vi "Time.vi"(8 "error in (no error)":errorcluster, 10 "Control In":T1={"I-O.lvclass"=refnum, "Gantry"=refnum, "Dispenser"="COM1"}, 11 "Sensor Dispense in":refnum<class "Sensor Dispense.lvclass">) -> (0 "error out":errorcluster, 1 "Timing Data":i32[](array[numeric]), 2 "Control Out":T1={"I-O.lvclass"=refnum, "Gantry"=refnum, "Dispenser"="COM1"}, 3 "Sensor Dispense out":refnum<class "Sensor Dispense.lvclass">)   [LabVIEW 2020, in "Sensor Dispense.lvclass"]
uses:
  Projects/Sensor Dispense.lvclass
  C:/Users/HEP/Documents/GitHub/UCSB-Gantry-HEP/Classes/Routine/Dispense/Dispense.lvclass
  Controller/Controllers.ctl
  Controller/I-O/I-O.lvclass
  C:/Program Files (x86)/Aerotech/A3200/LabVIEW/2010/Bin/Aerotech.A3200.dll
  Program Files (x86)/Aerotech/A3200/LabVIEW/2010/Bin/Aerotech.A3200.dll
  Projects/Sensor Dispense.lvclass/Sensor Dispense.ctl
  Controller/Motion/Motion.lvclass
  Controller/Motion/A3200/A3200.lvclass
  Controller/Controller.lvclass
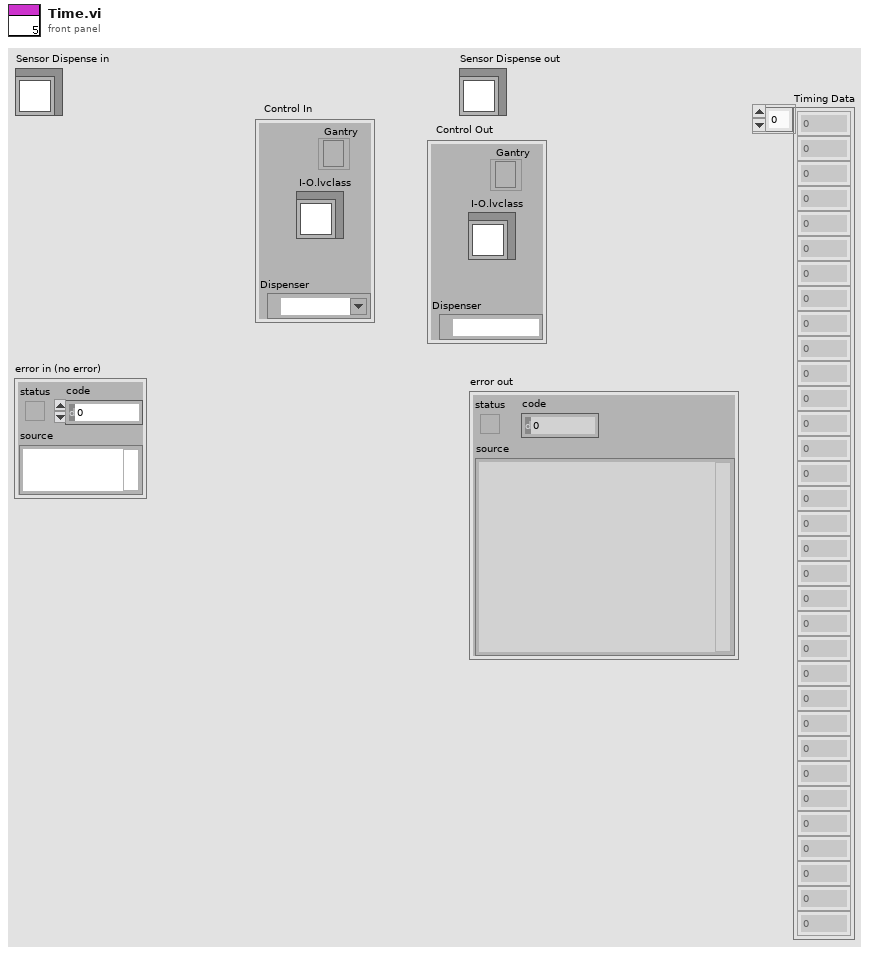
[diagram p1: front panel]
types:
  T1 = typedef "Controller.lvclass/Controllers.ctl" = cluster{"I-O.lvclass":refnum<class "I-O.lvclass">, "Gantry":refnum<k24>, "Dispenser":refnum<visa-resource-name>}
  T2 = cluster{"Endpoints":dbl[][], "Center":dbl[], "CW/CCW":dbl, "Dispense Type":enum16{"N-gon", "Square", "Arc", "Dot", "Line", "Circle"}}[]
  T3 = enum16{"N-gon", "Square", "Arc", "Dot", "Line", "Circle"}
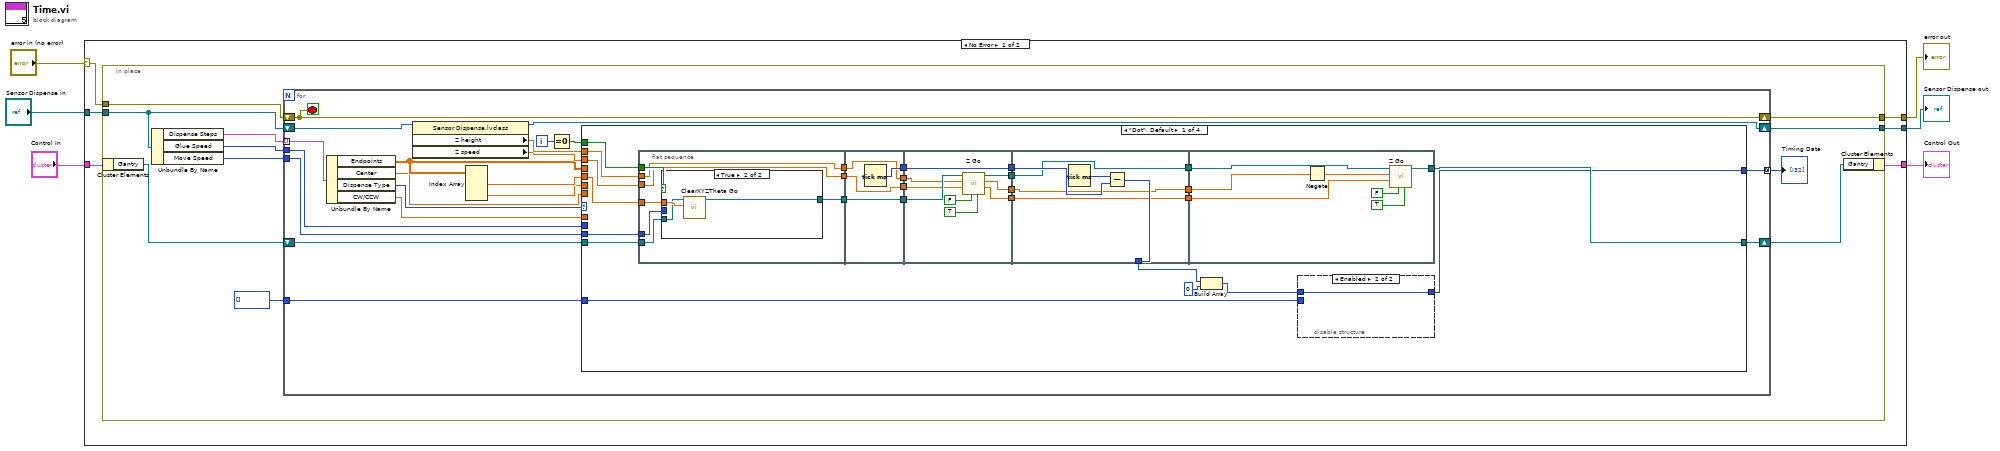
[diagram p0: block diagram]
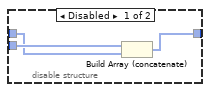
[diagram p2: hidden frame]
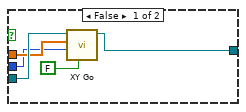
[diagram p3: hidden frame]
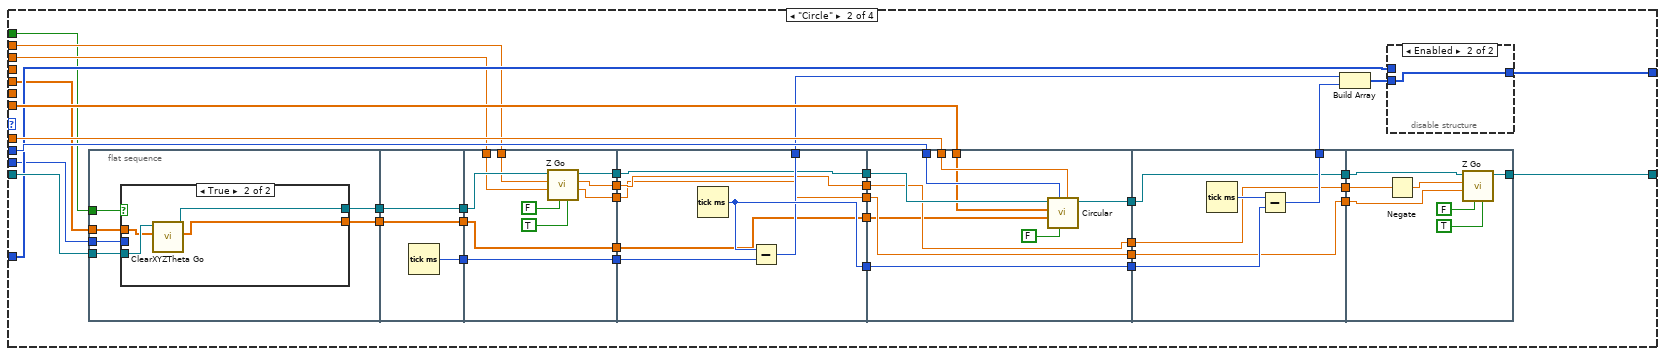
[diagram p4: hidden frame]
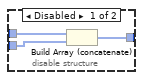
[diagram p5: hidden frame]
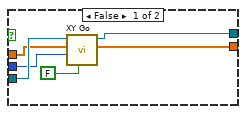
[diagram p6: hidden frame]
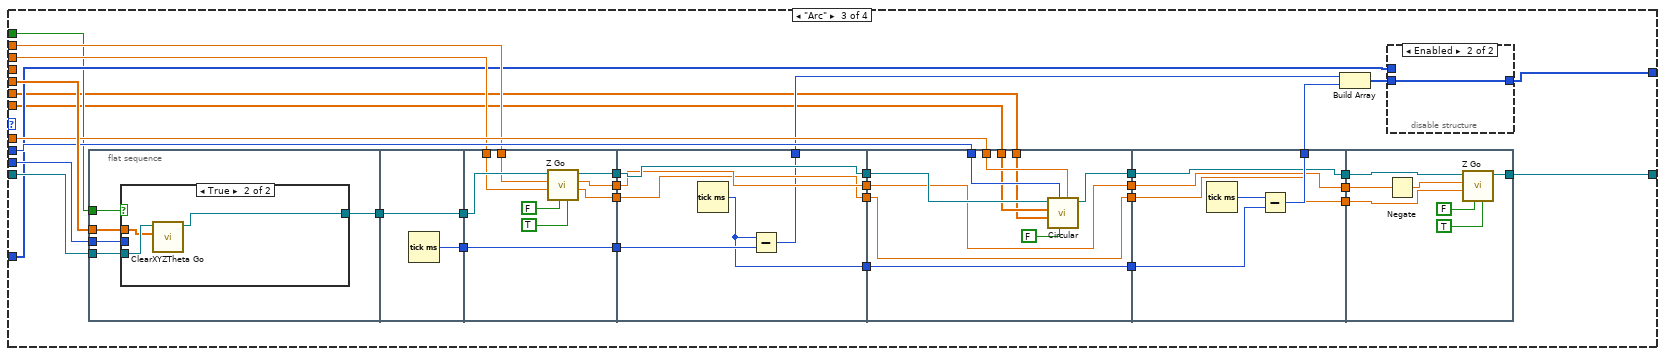
[diagram p7: hidden frame]
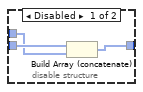
[diagram p8: hidden frame]
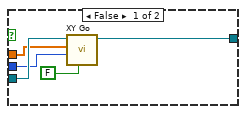
[diagram p9: hidden frame]
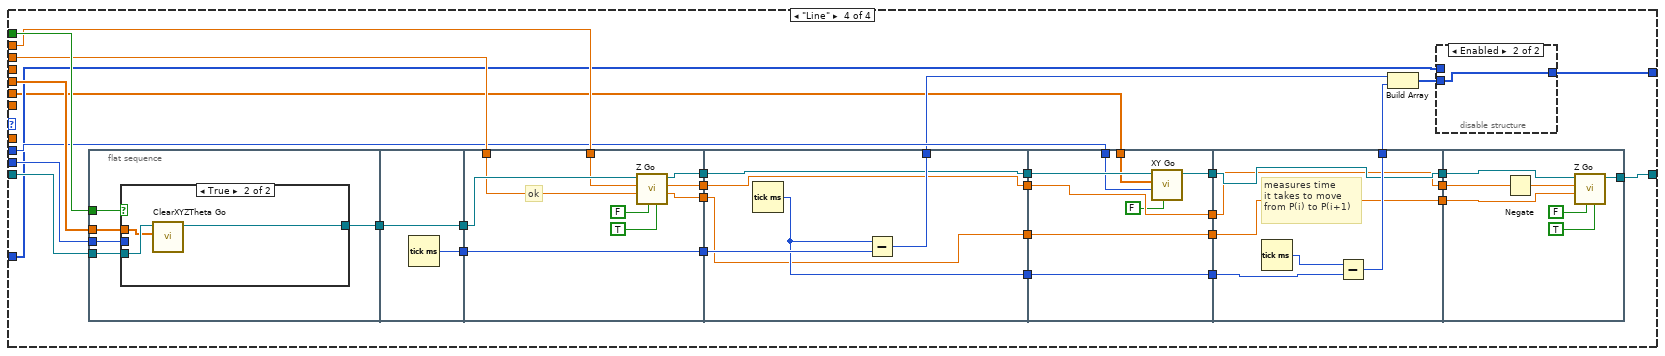
[diagram p10: hidden frame]
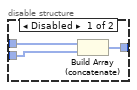
[diagram p11: hidden frame]
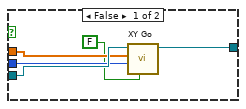
[diagram p12: hidden frame]
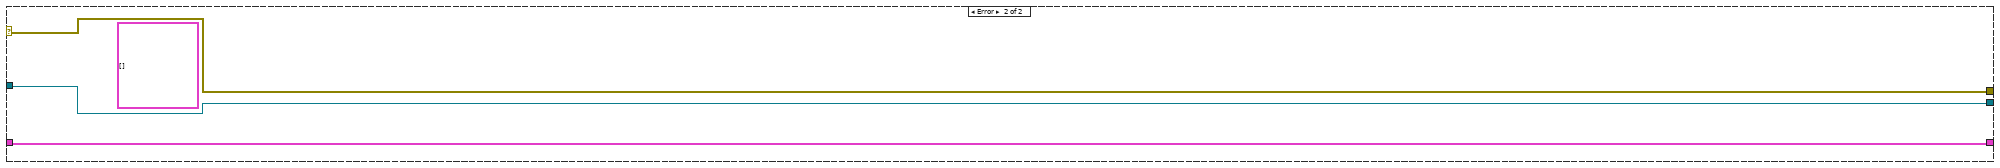
[diagram p13: hidden frame]
diagram:
  n1 = case shown="No Error" "error in (no error)" {
    selector: "error in (no error)" -> [w7 w395]
    tunnel: "Sensor Dispense in" -> [w12 w393]
    tunnel: [w11 w393] -> w5
    tunnel: "Control In" -> [w10 w394]
    tunnel: [w9 w394] -> w3
    tunnel: [w8 w395] -> w2
    frame No Error {
      n2 = in-place {
        in-place-border: w12 -> [w21]
        in-place-border: [w20] -> w11
        in-place-border: [w16] -> w8
        in-place-border: w7 -> [w15]
        n3 = in-place-cluster #1(w10) -> ("Gantry"=w22:refnum<k24>)
        n4 = Unbundle By Name "Unbundle By Name"(w21) -> ("Dispense Steps"=w17:T2, "Glue Speed"=w13:i32, "Move Speed"=w14:i32)
        n5 = for {
          tunnel: w14 -> [w43]
          shift-right: [w30] -> w19
          shift-left: w22 -> [w41]
          tunnel: w13 -> [w26]
          shift-right: [w39] -> w20
          shift-left: w21 -> [w40]
          tunnel: w17 -> [w33] mode=indexing
          shift-right: [w24] -> w16
          shift-left: w15 -> [w24]
          tunnel: i32[] [] -> [w42]
          tunnel: [w34] -> w18 mode=concatenating
          i -> [w38]
          stop <- w24 stop-if-true
          n6 = Unbundle By Name(w33) -> ("Endpoints"=w29:dbl[][], "Center"=w27:dbl[], "Dispense Type"=w32:T3, "CW/CCW"=w25:dbl)
          n7 = property class="Sensor Dispense.lvclass"(reference=w40) -> (reference out=w39:refnum<class "Sensor Dispense.lvclass">, "Z height"=w36:dbl, "Z speed"=w35:dbl)  [unwired: 1 in, 1 out]
          n8 = Index Array(array=w29) -> (element #1=w31:dbl[], element #2=w28:dbl[])  [unwired: 4 in]
          n9 = Equal To 0?(x=w38) -> (x = 0?=w37:bool)
          n10 = case shown="\"Dot\", Default" w32 {
            tunnel: w27 -> [_ w139 w223 _]
            tunnel: w41 -> [w65 w140 w248 w337]
            tunnel: w43 -> [w49 w128 w246 w335]
            tunnel: [w50 w147 w235 w311] -> w30
            tunnel: w26 -> [_ w138 w245 w325]
            tunnel: w25 -> [_ w137 w244 _]
            tunnel: w42 -> [w46 w134 w227 w309]
            tunnel: [w44 w132 w226 w307] -> w34
            tunnel: w31 -> [w66 w127 w247 w336]
            tunnel: w35 -> [w59 w130 w242 w330]
            tunnel: w36 -> [w62 w131 w243 w331]
            tunnel: w37 -> [w67 w129 w225 w334]
            tunnel: w29 -> [_ _ _ _]
            tunnel: w28 -> [_ _ w224 w306]
            frame "Dot", Default {
              n11 = flat-sequence {
                tunnel: w67 -> [w80]
                tunnel: w66 -> [w79]
                tunnel: w65 -> [w78]
                tunnel: [w77] -> w63
                tunnel: w62 -> [w76]
                tunnel: [w76] -> w60
                tunnel: w59 -> [w75]
                tunnel: [w75] -> w57
                tunnel: w49 -> [w74]
                tunnel: [w92] -> w69
                tunnel: [w91] -> w64
                tunnel: w63 -> [w91]
                tunnel: [w90] -> w61
                tunnel: w60 -> [w90]
                tunnel: [w89] -> w58
                tunnel: w57 -> [w89]
                tunnel: [w101] -> w68
                tunnel: w69 -> [w101]
                tunnel: w64 -> [w100]
                tunnel: w61 -> [w99]
                tunnel: w58 -> [w98]
                tunnel: [w97] -> w55
                tunnel: [w96] -> w53
                tunnel: [w95] -> w51
                tunnel: w68 -> [w107]
                tunnel: [w105] -> w48
                tunnel: [w104] -> w56
                tunnel: w55 -> [w104]
                tunnel: [w103] -> w54
                tunnel: w53 -> [w103]
                tunnel: [w102] -> w52
                tunnel: w51 -> [w102]
                tunnel: w56 -> [w114]
                tunnel: w54 -> [w112]
                tunnel: w52 -> [w111]
                tunnel: [w110] -> w50
                frame #0 {
                  n12 = case shown="True" w80 {
                    tunnel: w79 -> [w83 w88]
                    tunnel: w78 -> [w85 w87]
                    tunnel: [w84 w86] -> w77
                    tunnel: w74 -> [w82 _]
                    frame False {
                      n13 = call "XY Go.vi"("return immediately"=FALSE, "Speed"=w82, "XY In"=w83, "Gantry In"=w85) -> ("Gantry Out"=w84:refnum<k24>)  [unwired: 5 in, 2 out]
                    }
                    frame True {
                      n14 = call "ClearXYZTheta Go.vi"("XYZTheta In"=w88, "Gantry In"=w87) -> ("Gantry Out"=w86:refnum<k24>)  [unwired: 7 in, 2 out]
                    }
                  }
                }
                frame #1 {
                  n15 = Tick Count (ms)() -> (millisecond timer value=w92:u32)
                }
                frame #2 {
                  n16 = call "Z Go.vi"("Increment"=TRUE, "Return Immediately"=FALSE, "Speed In"=w98, "Position In"=w99, "Gantry In"=w100) -> ("Speed Out"=w96:dbl, "Position Out"=w97:dbl, "Gantry Out"=w95:refnum<k24>)  [unwired: 3 in, 1 out]
                }
                frame #3 {
                  n17 = Tick Count (ms)() -> (millisecond timer value=w106:u32)
                  n18 = Subtract(x=w106, y=w107) -> (x-y=w105:u32)
                }
                frame #4 {
                  n19 = Negate(x=w114) -> (-x=w113:dbl)
                  n20 = call "Z Go.vi"("Increment"=TRUE, "Return Immediately"=FALSE, "Speed In"=w112, "Position In"=w113, "Gantry In"=w111) -> ("Gantry Out"=w110:refnum<k24>)  [unwired: 3 in, 3 out]
                }
              }
              n21 = Build Array(w48, u32 0 ("element")) -> (w45:u32[])
              n22 = disable-structure shown="Enabled" {
                disable-tunnel: w46 -> [w72 _]
                disable-tunnel: w45 -> [w71 w73]
                disable-tunnel: [w70 w73] -> w44
                frame Disabled {
                  n23 = Build Array (concatenate)(w72, w71) -> (w70:u32[])
                }
                frame Enabled {
                }
              }
            }
            frame "Circle" {
              n24 = flat-sequence {
                tunnel: [w158] -> w145
                tunnel: w140 -> [w159]
                tunnel: w127 -> [w160]
                tunnel: w129 -> [w161]
                tunnel: w128 -> [w157]
                tunnel: [w156] -> w123
                tunnel: [w174] -> w151
                tunnel: [w173] -> w146
                tunnel: w145 -> [w173]
                tunnel: [w172] -> w124
                tunnel: w123 -> [w172]
                tunnel: w151 -> [w184]
                tunnel: [w184] -> w150
                tunnel: w146 -> [w182]
                tunnel: [w181] -> w144
                tunnel: w131 -> [w180]
                tunnel: w130 -> [w179]
                tunnel: [w183] -> w125
                tunnel: w124 -> [w183]
                tunnel: [w178] -> w120
                tunnel: [w177] -> w117
                tunnel: w150 -> [w191]
                tunnel: [w190] -> w148
                tunnel: [w189] -> w136
                tunnel: w144 -> [w188]
                tunnel: [w188] -> w143
                tunnel: [w187] -> w126
                tunnel: w125 -> [w187]
                tunnel: [w186] -> w121
                tunnel: w120 -> [w186]
                tunnel: [w185] -> w118
                tunnel: w117 -> [w185]
                tunnel: [w201] -> w149
                tunnel: w148 -> [w201]
                tunnel: w143 -> [w200]
                tunnel: [w199] -> w141
                tunnel: w139 -> [w193]
                tunnel: w138 -> [w198]
                tunnel: w137 -> [w195]
                tunnel: w126 -> [w194]
                tunnel: [w197] -> w122
                tunnel: w121 -> [w197]
                tunnel: [w196] -> w119
                tunnel: w118 -> [w196]
                tunnel: w149 -> [w206]
                tunnel: [w205] -> w135
                tunnel: [w204] -> w142
                tunnel: w141 -> [w204]
                tunnel: w122 -> [w203]
                tunnel: w119 -> [w202]
                tunnel: [w203] -> w116
                tunnel: [w202] -> w115
                tunnel: [w212] -> w147
                tunnel: w142 -> [w213]
                tunnel: w116 -> [w214]
                tunnel: w115 -> [w211]
                frame #0 {
                  n25 = case shown="True" w161 {
                    tunnel: w160 -> [w162 w169]
                    tunnel: w159 -> [w167 w171]
                    tunnel: [w166 w170] -> w158
                    tunnel: w157 -> [w165 _]
                    tunnel: [w164 w168] -> w156
                    frame False {
                      n26 = call "XY Go.vi"("return immediately"=FALSE, "Speed"=w165, "XY In"=w162, "Gantry In"=w167) -> ("XY Out"=w164:dbl[], "Gantry Out"=w166:refnum<k24>)  [unwired: 5 in, 1 out]
                    }
                    frame True {
                      n27 = call "ClearXYZTheta Go.vi"("XYZTheta In"=w169, "Gantry In"=w171) -> ("XYZTheta Out"=w168:dbl[], "Gantry Out"=w170:refnum<k24>)  [unwired: 7 in, 1 out]
                    }
                  }
                }
                frame #1 {
                  n28 = Tick Count (ms)() -> (millisecond timer value=w174:u32)
                }
                frame #2 {
                  n29 = call "Z Go.vi"("Increment"=TRUE, "Return Immediately"=FALSE, "Speed In"=w179, "Position In"=w180, "Gantry In"=w182) -> ("Speed Out"=w177:dbl, "Position Out"=w178:dbl, "Gantry Out"=w181:refnum<k24>)  [unwired: 3 in, 1 out]
                }
                frame #3 {
                  n30 = Tick Count (ms)() -> (millisecond timer value=w190:u32)
                  n31 = Subtract(x=w190, y=w191) -> (x-y=w189:u32)
                }
                frame #4 {
                  n32 = call "Circular.vi"("Direction"=w195, "return immediately"=FALSE, "Speed"=w198, "XY End"=w194, "XY Center"=w193, "Gantry In"=w200) -> ("Gantry Out"=w199:refnum<k24>)  [unwired: 4 in, 1 out]
                }
                frame #5 {
                  n33 = Tick Count (ms)() -> (millisecond timer value=w207:u32)
                  n34 = Subtract(x=w207, y=w206) -> (x-y=w205:u32)
                }
                frame #6 {
                  n35 = Negate(x=w214) -> (-x=w210:dbl)
                  n36 = call "Z Go.vi"("Increment"=TRUE, "Return Immediately"=FALSE, "Speed In"=w211, "Position In"=w210, "Gantry In"=w213) -> ("Gantry Out"=w212:refnum<k24>)  [unwired: 3 in, 3 out]
                }
              }
              n37 = Build Array(w136, w135) -> (w133:u32[])
              n38 = disable-structure shown="Enabled" {
                disable-tunnel: w134 -> [w154 _]
                disable-tunnel: w133 -> [w153 w155]
                disable-tunnel: [w152 w155] -> w132
                frame Disabled {
                  n39 = Build Array (concatenate)(w154, w153) -> (w152:u32[])
                }
                frame Enabled {
                }
              }
            }
            frame "Arc" {
              n40 = flat-sequence {
                tunnel: w248 -> [w257]
                tunnel: w247 -> [w256]
                tunnel: w246 -> [w255]
                tunnel: [w254] -> w239
                tunnel: w225 -> [w253]
                tunnel: w239 -> [w267]
                tunnel: [w267] -> w238
                tunnel: [w266] -> w236
                tunnel: w238 -> [w276]
                tunnel: [w273] -> w241
                tunnel: w243 -> [w275]
                tunnel: w242 -> [w274]
                tunnel: [w272] -> w237
                tunnel: w236 -> [w272]
                tunnel: [w271] -> w233
                tunnel: [w270] -> w231
                tunnel: w241 -> [w282]
                tunnel: [w282] -> w240
                tunnel: w237 -> [w281]
                tunnel: [w280] -> w234
                tunnel: w233 -> [w280]
                tunnel: [w279] -> w232
                tunnel: w231 -> [w279]
                tunnel: [w278] -> w230
                tunnel: [w277] -> w216
                tunnel: w240 -> [w292]
                tunnel: w245 -> [w291]
                tunnel: w244 -> [w290]
                tunnel: w234 -> [w286]
                tunnel: w232 -> [w285]
                tunnel: w223 -> [w289]
                tunnel: w224 -> [w288]
                tunnel: [w287] -> w221
                tunnel: [w286] -> w219
                tunnel: [w285] -> w217
                tunnel: w216 -> [w284]
                tunnel: [w284] -> w215
                tunnel: [w298] -> w229
                tunnel: [w297] -> w222
                tunnel: w221 -> [w297]
                tunnel: [w296] -> w220
                tunnel: w219 -> [w296]
                tunnel: [w295] -> w218
                tunnel: w217 -> [w295]
                tunnel: w215 -> [w293]
                tunnel: [w305] -> w235
                tunnel: w222 -> [w303]
                tunnel: w220 -> [w302]
                tunnel: w218 -> [w301]
                frame #0 {
                  n41 = case shown="True" w253 {
                    tunnel: [w262 w265] -> w254
                    tunnel: w257 -> [w261 w264]
                    tunnel: w256 -> [w258 w263]
                    tunnel: w255 -> [w260 _]
                    frame False {
                      n42 = call "XY Go.vi"("return immediately"=FALSE, "Speed"=w260, "XY In"=w258, "Gantry In"=w261) -> ("Gantry Out"=w262:refnum<k24>)  [unwired: 5 in, 2 out]
                    }
                    frame True {
                      n43 = call "ClearXYZTheta Go.vi"("XYZTheta In"=w263, "Gantry In"=w264) -> ("Gantry Out"=w265:refnum<k24>)  [unwired: 7 in, 2 out]
                    }
                  }
                }
                frame #1 {
                  n44 = Tick Count (ms)() -> (millisecond timer value=w266:u32)
                }
                frame #2 {
                  n45 = call "Z Go.vi"("Increment"=TRUE, "Return Immediately"=FALSE, "Speed In"=w274, "Position In"=w275, "Gantry In"=w276) -> ("Speed Out"=w270:dbl, "Position Out"=w271:dbl, "Gantry Out"=w273:refnum<k24>)  [unwired: 3 in, 1 out]
                }
                frame #3 {
                  n46 = Tick Count (ms)() -> (millisecond timer value=w277:u32)
                  n47 = Subtract(x=w277, y=w281) -> (x-y=w278:u32)
                }
                frame #4 {
                  n48 = call "Circular.vi"("Direction"=w290, "return immediately"=FALSE, "Speed"=w291, "XY End"=w288, "XY Center"=w289, "Gantry In"=w292) -> ("Gantry Out"=w287:refnum<k24>)  [unwired: 4 in, 1 out]
                }
                frame #5 {
                  n49 = Tick Count (ms)() -> (millisecond timer value=w294:u32)
                  n50 = Subtract(x=w294, y=w293) -> (x-y=w298:u32)
                }
                frame #6 {
                  n51 = Negate(x=w302) -> (-x=w304:dbl)
                  n52 = call "Z Go.vi"("Increment"=TRUE, "Return Immediately"=FALSE, "Speed In"=w301, "Position In"=w304, "Gantry In"=w303) -> ("Gantry Out"=w305:refnum<k24>)  [unwired: 3 in, 3 out]
                }
              }
              n53 = Build Array(w230, w229) -> (w228:u32[])
              n54 = disable-structure shown="Enabled" {
                disable-tunnel: w228 -> [w251 w252]
                disable-tunnel: w227 -> [w250 _]
                disable-tunnel: [w249 w252] -> w226
                frame Disabled {
                  n55 = Build Array (concatenate)(w251, w250) -> (w249:u32[])
                }
                frame Enabled {
                }
              }
            }
            frame "Line" {
              n56 = flat-sequence {
                tunnel: w337 -> [w346]
                tunnel: w336 -> [w342]
                tunnel: w335 -> [w345]
                tunnel: w334 -> [w344]
                tunnel: [w343] -> w333
                tunnel: w333 -> [w355]
                tunnel: [w355] -> w332
                tunnel: [w356] -> w328
                tunnel: w332 -> [w365]
                tunnel: w331 -> [w364]
                tunnel: w330 -> [w363]
                tunnel: [w362] -> w329
                tunnel: w328 -> [w362]
                tunnel: [w361] -> w326
                tunnel: [w360] -> w317
                tunnel: [w359] -> w313
                tunnel: w329 -> [w371]
                tunnel: [w370] -> w310
                tunnel: [w369] -> w327
                tunnel: w326 -> [w369]
                tunnel: [w368] -> w323
                tunnel: [w367] -> w318
                tunnel: w317 -> [w367]
                tunnel: [w366] -> w314
                tunnel: w313 -> [w366]
                tunnel: w327 -> [w379]
                tunnel: w325 -> [w378]
                tunnel: [w377] -> w324
                tunnel: w323 -> [w377]
                tunnel: [w376] -> w321
                tunnel: [w375] -> w319
                tunnel: w318 -> [w375]
                tunnel: [w374] -> w315
                tunnel: w314 -> [w374]
                tunnel: w306 -> [w373]
                tunnel: w324 -> [w384]
                tunnel: [w383] -> w312
                tunnel: [w382] -> w322
                tunnel: w321 -> [w382]
                tunnel: [w381] -> w320
                tunnel: w319 -> [w381]
                tunnel: [w380] -> w316
                tunnel: w315 -> [w380]
                tunnel: w322 -> [w392]
                tunnel: w320 -> [w391]
                tunnel: w316 -> [w389]
                tunnel: [w388] -> w311
                frame #0 {
                  n57 = case shown="True" w344 {
                    tunnel: w346 -> [w351 w354]
                    tunnel: w345 -> [w350 _]
                    tunnel: [w349 w353] -> w343
                    tunnel: w342 -> [w348 w352]
                    frame False {
                      n58 = call "XY Go.vi"("return immediately"=FALSE, "Speed"=w350, "XY In"=w348, "Gantry In"=w351) -> ("Gantry Out"=w349:refnum<k24>)  [unwired: 5 in, 2 out]
                    }
                    frame True {
                      n59 = call "ClearXYZTheta Go.vi"("XYZTheta In"=w352, "Gantry In"=w354) -> ("Gantry Out"=w353:refnum<k24>)  [unwired: 7 in, 2 out]
                    }
                  }
                }
                frame #1 {
                  n60 = Tick Count (ms)() -> (millisecond timer value=w356:u32)
                }
                frame #2 {
                  # "ok"
                  n61 = call "Z Go.vi"("Increment"=TRUE, "Return Immediately"=FALSE, "Speed In"=w363, "Position In"=w364, "Gantry In"=w365) -> ("Speed Out"=w359:dbl, "Position Out"=w360:dbl, "Gantry Out"=w361:refnum<k24>)  [unwired: 3 in, 1 out]
                }
                frame #3 {
                  n62 = Tick Count (ms)() -> (millisecond timer value=w368:u32)
                  n63 = Subtract(x=w368, y=w371) -> (x-y=w370:u32)
                }
                frame #4 {
                  n64 = call "XY Go.vi"("return immediately"=FALSE, "Speed"=w378, "XY In"=w373, "Gantry In"=w379) -> ("Gantry Out"=w376:refnum<k24>)  [unwired: 5 in, 2 out]
                }
                frame #5 {
                  # "measures time\nit takes to move\nfrom P(i) to P(i+1)"
                  n65 = Tick Count (ms)() -> (millisecond timer value=w385:u32)
                  n66 = Subtract(x=w385, y=w384) -> (x-y=w383:u32)
                }
                frame #6 {
                  n67 = Negate(x=w391) -> (-x=w390:dbl)
                  n68 = call "Z Go.vi"("Increment"=TRUE, "Return Immediately"=FALSE, "Speed In"=w389, "Position In"=w390, "Gantry In"=w392) -> ("Gantry Out"=w388:refnum<k24>)  [unwired: 3 in, 3 out]
                }
              }
              n69 = Build Array(w310, w312) -> (w308:u32[])
              n70 = disable-structure shown="Enabled" {
                disable-tunnel: w309 -> [w340 _]
                disable-tunnel: w308 -> [w339 w341]
                disable-tunnel: [w338 w341] -> w307
                frame Disabled {
                  n71 = Build Array (concatenate)(w340, w339) -> (w338:u32[])
                }
                frame Enabled {
                }
              }
            }
          }
        }
        "Timing Data" <- w18
        n72 = in-place-cluster #1("Gantry"=w19) -> (w9:T1)
      }
    }
    frame Error {
      (unwired) T2 [] ("Dispense Steps")
    }
  }
  "error out" <- w2
  "Sensor Dispense out" <- w5
  "Control Out" <- w3
